vi "Autonomous Independent.vi"() -> ()   [LabVIEW 2017]
doc: "This VI is called when autonomous begins, and will automatically be terminated when autonomous ends. You can carry out timed or sensor driven robot movement independently without needing to return to the caller."
uses:
  Motion_Profiler_Class/MotionProfiles.lvclass
  <vilib>/Rock Robotics/WPI/Utilities/WPI_GetSetVariantRefNum.vi
  <vilib>/Rock Robotics/Network Tables/NT Read String.vi
  <vilib>/Rock Robotics/Network Tables/NT Write Numeric Array.vi
panel:
  out "Left Motor":T1(graph)
  out "Left Throttle":dbl(graph)
  out "Right Motor":T1(graph)
  out "Right Throttle":dbl(graph)
  out "Right Prof Count":i32
  out "Left Prof Count":i32
  out "Mot Prof Active Is Under Run":bool
  in  "?":bool
  # "Be sure to right-click and choose Data Operations>>Make Current Value default if you want to save the array values with the VI"
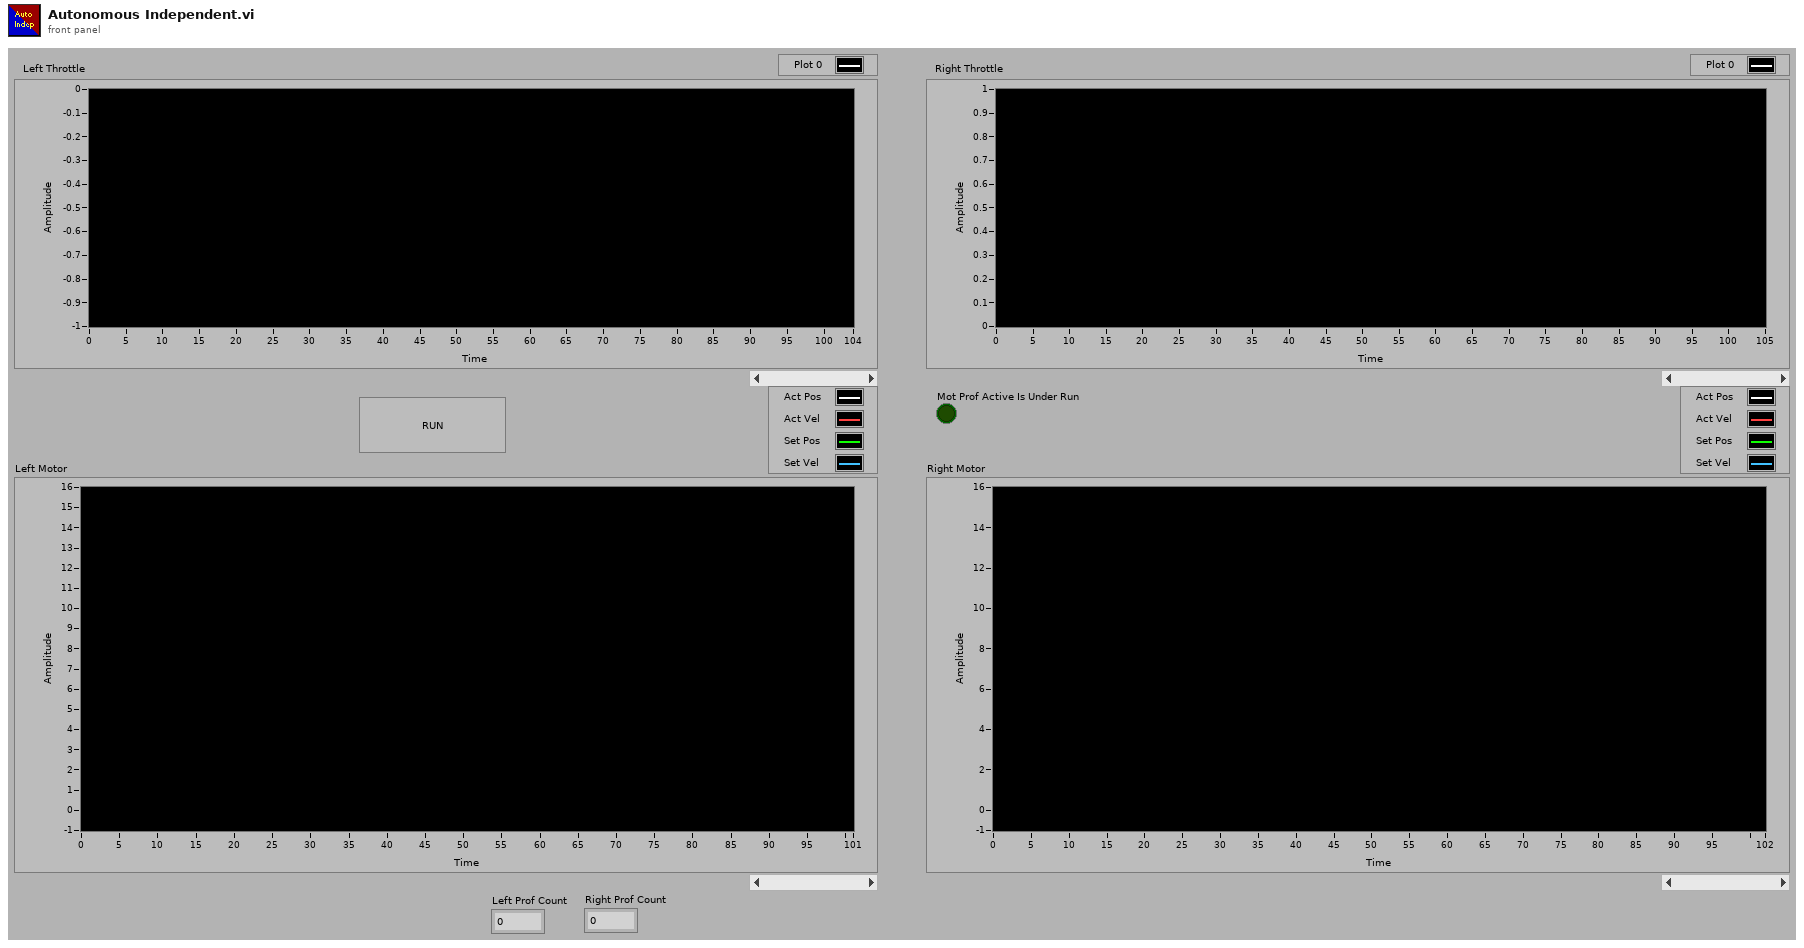
[diagram p1: front panel]
types:
  T1 = cluster{"Sensor Position":dbl, "Sensor Velocity":dbl, "Mot Prof Active Position":dbl, "Mot Prof Active Velocity":dbl}
  T2 = typedef "WPI_JoystickDevRef.ctl" = cluster{"Device":T3}
  T3 = typedef "WPI_JoystickDeviceEnum.ctl" = enum16{"USB 0", "USB 1", "USB 2", "USB 3", "USB 4", "USB 5"}
  T4 = typedef "WPI_MotorControlDeviceRef.ctl" = cluster{"DeviceStatus":errorcluster, "Type":T5, "PWM":cluster{"PWM Channel":T6, "DeadBand":T7}, "CAN":cluster{"Device Number":u8, "SetOutput VI Ref":variant, "GetOutput VI Ref":variant, "Enable VI Ref":variant, "Disable VI Ref":variant, "Data":variant}, "Invert":bool, "DIO PWM":cluster{"PWM \"Enable\" Channel":T6, "DIOChannel":T8, "PWM Rate":dbl}}
  T5 = typedef "WPI_MotorControlType.ctl" = enum16{"PWM", "CAN", "DIO PWM"}
  T6 = typedef "FPGA_DIOPWMChannel.ctl" = enum8{"PWM 0", "PWM 1", "PWM 2", "PWM 3", "PWM 4", "PWM 5", "PWM 6", "PWM 7", "PWM 8", "PWM 9", "PWM MXP 0", "PWM MXP 1", "PWM MXP 2", "PWM MXP 3", "PWM MXP 4", "PWM MXP 5", "PWM MXP 6", "PWM MXP 7", "PWM MXP 8", "PWM MXP 9", "Invalid"}
  T7 = typedef "WPI_PWMDeadband.ctl" = cluster{"Name":string, "maxPositivePwm":i32, "minPositivePwm":i32, "centerPwm":i32, "maxNegativePwm":i32, "minNegativePwm":i32, "angularRange":u16}
  T8 = typedef "FPGA_DIOChannel.ctl" = enum8{"DIO 0", "DIO 1", "DIO 2", "DIO 3", "DIO 4", "DIO 5", "DIO 6", "DIO 7", "DIO 8", "DIO 9", "DIO MXP 0", "DIO MXP 1", "DIO MXP 2", "DIO MXP 3", "DIO MXP 4", "DIO MXP 5", "DIO MXP 6", "DIO MXP 7", "DIO MXP 8", "DIO MXP 9", "DIO MXP 10", "DIO MXP 11", "DIO MXP 12", "DIO MXP 13", "DIO MXP 14", "DIO MXP 15", "SPI Port CS1", "SPI Port CS2", "SPI Port CS3", "SPI Port MISO", "SPI Port MOSI", "Invalid"}
  T9 = cluster{"Top Buffer Remaining":i32, "Top Buffer Count":i32, "Bottom Buffer Count":i32, "Has Underrun?":bool, "Is Underrun?":bool, "Active Point Valid?":bool, "Is Last?":bool, "Profile Slot Select 0":i32, "Output Enable":i32, "Time Duration (ms)":i32, "Profile Slot Select 1":i32}
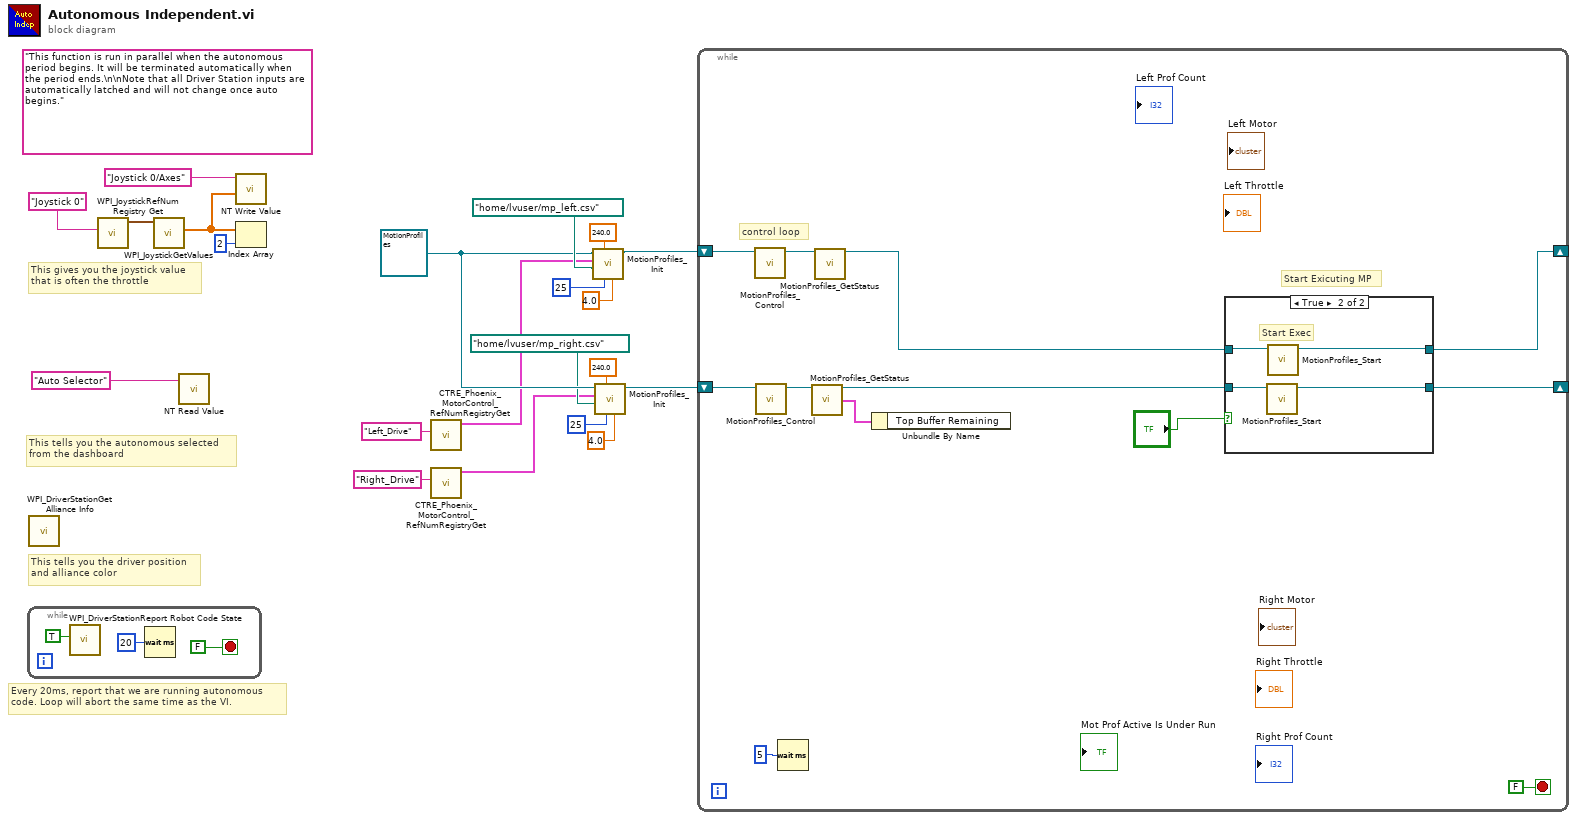
[diagram p0: block diagram]
diagram:
  w11 = refnum<class "MotionProfiles.lvclass"> refnum ("MotionProfiles.lvclass")
  (unwired) "This function is run in parallel when the autonomous period begins. It will be terminated automatically when the period ends.\n\nNote that all Driver Station inputs are automatically latched and will not change once auto begins."
  # "This tells you the autonomous selected\nfrom the dashboard"
  # "Every 20ms, report that we are running autonomous\ncode. Loop will abort the same time as the VI."
  # "This gives you the joystick value\nthat is often the throttle"
  # "This tells you the driver position\nand alliance color"
  n1 = while {
    stop <- FALSE stop-if-true
    n2 = call <vilib>:"WPI_DriverStationReport Robot Code State.vi"("Autonomous"=TRUE) -> ()  [unwired: 10 in, 1 out]
    n3 = Wait (ms)(milliseconds to wait=u32 20) -> ()  [unwired: 1 out]
  }
  n4 = call <vilib>:"WPI_DriverStationGet Alliance Info.vi"() -> ()  [unwired: 12 out]
  n5 = call <vilib>:"WPI_JoystickRefNum Registry Get.vi"("refnum name"="Joystick 0") -> ("JoystickDevRef"=w20:T2)  [unwired: 1 in, 9 out]
  n6 = call <vilib>:"WPI_JoystickGetValues.vi"("JoystickDevRef"=w20) -> ("Axes"=w17:dbl[])  [unwired: 6 in, 4 out]
  n7 = call-poly <vilib>:"NT Read Value.vi"("Name"="Auto Selector") -> ()  [unwired: 9 in, 2 out]
  n8 = call-poly <vilib>:"NT Write Value.vi"("Numeric Array"=w17, "Name"="Joystick 0/Axes") -> ()  [unwired: 9 in, 1 out]
  n9 = Index Array(array=w17, index=2) -> ()  [unwired: 1 out]
  n10 = call <vilib>:"CTRE_Phoenix_MotorControl_RefNumRegistryGet.vi"("refnum name"="Left_Drive") -> ("PhoenixMotorControlDevRef"=w6:T4)  [unwired: 9 in, 1 out]
  n11 = call <vilib>:"CTRE_Phoenix_MotorControl_RefNumRegistryGet.vi"("refnum name"="Right_Drive") -> ("PhoenixMotorControlDevRef"=w7:T4)  [unwired: 9 in, 1 out]
  n12 = call "MotionProfiles_Init.vi"("Wheel_Diameter (in)"=4.0 ("Wheel Diameter"), "MP_Frame_Rate_(ms)"=25, "Encoder_CPR_4x"=240.0, "CSV File Path"=path "/home/lvuser/mp_left.csv" ("file path (use dialog)"), "PhoenixMotorControlDevRef"=w6, "MotionProfiles in"=w11) -> ("MotionProfiles out"=w15:refnum<class "MotionProfiles.lvclass">)  [unwired: 4 in, 1 out]
  n13 = call "MotionProfiles_Init.vi"("Wheel_Diameter (in)"=4.0, "MP_Frame_Rate_(ms)"=25, "Encoder_CPR_4x"=240.0, "CSV File Path"=path "/home/lvuser/mp_right.csv" ("file path (use dialog)"), "PhoenixMotorControlDevRef"=w7, "MotionProfiles in"=w11) -> ("MotionProfiles out"=w12:refnum<class "MotionProfiles.lvclass">)  [unwired: 4 in, 1 out]
  n14 = while {
    shift-right: [w31] -> _
    shift-left: w15 -> [w34]
    shift-right: [w32] -> _
    shift-left: w12 -> [w33]
    stop <- FALSE stop-if-true
    # "control loop"
    # "Start Exicuting MP"
    n15 = call "MotionProfiles_Control.vi"("MotionProfiles in"=w34) -> ("MotionProfiles out"=w28:refnum<class "MotionProfiles.lvclass">)  [unwired: 9 in, 1 out]
    n16 = call "MotionProfiles_Control.vi"("MotionProfiles in"=w33) -> ("MotionProfiles out"=w27:refnum<class "MotionProfiles.lvclass">)  [unwired: 9 in, 1 out]
    n17 = Wait (ms)(milliseconds to wait=u32 5) -> ()  [unwired: 1 out]
    n18 = call "MotionProfiles_GetStatus.vi"("MotionProfiles in"=w27) -> ("MotionProfiles out"=w29:refnum<class "MotionProfiles.lvclass">, "Motion Profile Status"=w25:T9)  [unwired: 9 in, 4 out]
    n19 = call "MotionProfiles_GetStatus.vi"("MotionProfiles in"=w28) -> ("MotionProfiles out"=w30:refnum<class "MotionProfiles.lvclass">)  [unwired: 9 in, 5 out]
    n20 = Unbundle By Name(w25) -> ()  [unwired: 1 out]
    n21 = case shown="True" "?" {
      tunnel: w30 -> [w38 w42]
      tunnel: w29 -> [w37 w40]
      tunnel: [w37 w39] -> w32
      tunnel: [w38 w41] -> w31
      frame False {
      }
      frame True {
        # "Start Exec"
        n22 = call "MotionProfiles_Start.vi"("MotionProfiles in"=w40) -> ("MotionProfiles out"=w39:refnum<class "MotionProfiles.lvclass">)  [unwired: 9 in, 1 out]
        n23 = call "MotionProfiles_Start.vi"("MotionProfiles in"=w42) -> ("MotionProfiles out"=w41:refnum<class "MotionProfiles.lvclass">)  [unwired: 9 in, 1 out]
      }
    }
  }
